vi "Write Log Session.vi"(8 "error in (no error)":errorcluster, 10 "Session Handle":T1, 11 "Network Actor in":refnum<class "Network Actor.lvclass">) -> (0 "error out":errorcluster, 3 "Network Actor out":refnum<class "Network Actor.lvclass">)   [LabVIEW 2014, in "Network Actor Library.lvlib" / "Network Actor.lvclass"]
uses:
  Network Actor.lvclass
  <userlib>/_Session Fwk/Typedefs/Session Handle.ctl
  <userlib>/_Session Fwk/Session - Root.lvclass
  Network Actor.lvclass/Network Actor.ctl
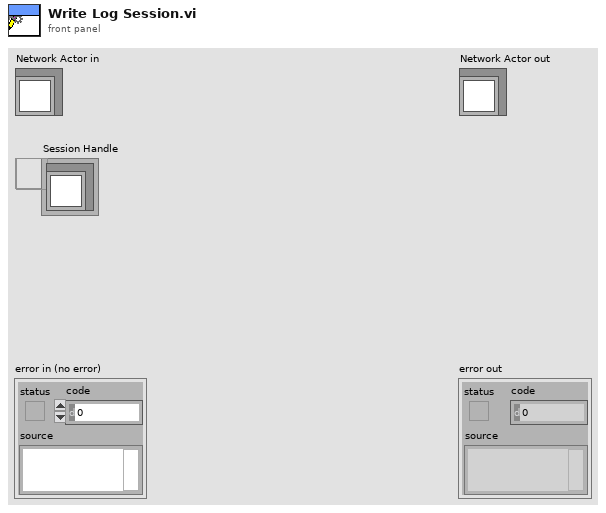
[diagram p1: front panel]
types:
  T1 = typedef "Session - Root.lvclass/Session Handle.ctl" = refnum<data-value>
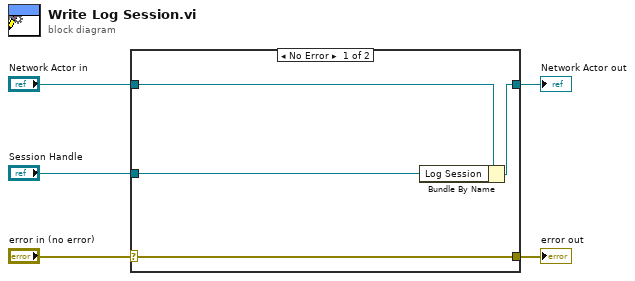
[diagram p0: block diagram]
diagram:
  n1 = case shown="No Error" "error in (no error)" {
    selector: "error in (no error)" -> [w9 w10]
    tunnel: [w9 w10] -> w4
    tunnel: [w7 w11] -> w2
    tunnel: "Network Actor in" -> [w8 w11]
    tunnel: "Session Handle" -> [w6 _]
    frame No Error {
      n2 = Bundle By Name(cluster=w8, "Log Session"=w6) -> (w7:refnum<class "Network Actor.lvclass">)
    }
    frame Error {
    }
  }
  "error out" <- w4
  "Network Actor out" <- w2
